vi "control_thor_z825b.vi"() -> ()   [LabVIEW 2013]
panel:
  out "error out":errorcluster
  out "pfPosition":sgl
  in  "stop":bool
  in  "serial":i32
  in  "MG17Motor":refnum<k7>(container)
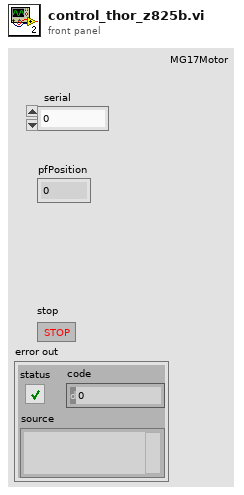
[diagram p1: front panel]
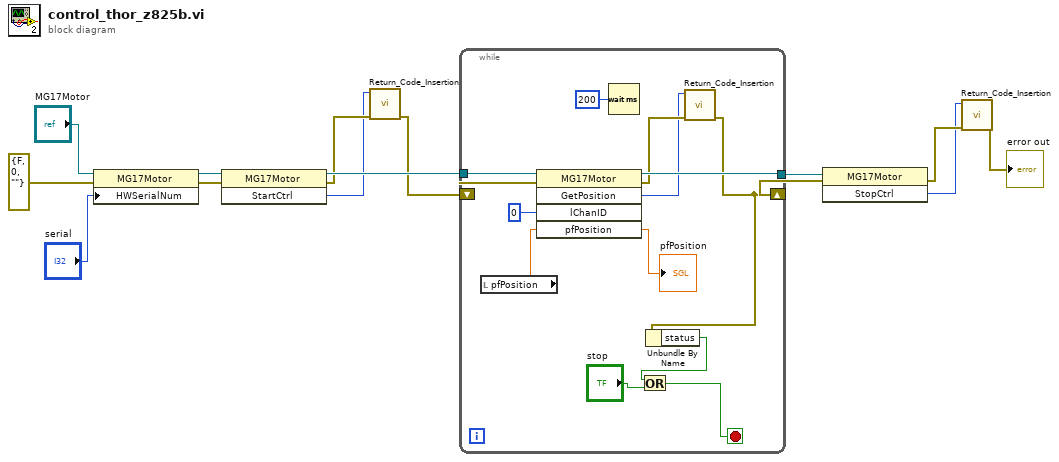
[diagram p0: block diagram]
diagram:
  n1 = property class="MG17Motor"(reference="MG17Motor", error in=errorcluster {"status"=FALSE, "code"=0, "source"=""} ("error in (no error)"), "HWSerialNum"="serial") -> (reference out=w12:refnum<k7>, error out=w8:errorcluster)
  n2 = invoke class="MG17Motor" method="StartCtrl"(reference=w12, error in=w8) -> (reference out=w11:refnum<k7>, error out=w7:errorcluster, "StartCtrl"=w6:i32)  [unwired: 1 in]
  n3 = call "Return_Code_Insertion.vi"("error in (no error)"=w7, "Return Code"=w6) -> ("error out"=w5:errorcluster)  [unwired: 9 in]
  n4 = while {
    tunnel: w11 -> [w27]
    tunnel: [w26] -> w10
    shift-right: [w18] -> w4
    shift-left: w5 -> [w21]
    stop <- w15 stop-if-true
    n5 = local read "pfPosition"() -> (w23:sgl)
    n6 = invoke class="MG17Motor" method="GetPosition"(reference=w27, error in=w21, "lChanID"=0, "pfPosition"=w23) -> (reference out=w26:refnum<k7>, error out=w20:errorcluster, "GetPosition"=w19:i32, "pfPosition"=→"pfPosition":sgl)  [unwired: 1 in, 1 out]
    n7 = Wait (ms)(milliseconds to wait=u32 200) -> ()  [unwired: 1 out]
    n8 = call "Return_Code_Insertion.vi"("error in (no error)"=w20, "Return Code"=w19) -> ("error out"=w18:errorcluster)  [unwired: 9 in]
    n9 = Unbundle By Name(w18) -> ("status"=w17:bool)
    n10 = Or(x=w17, y="stop") -> (x .or. y?=w15:bool)
  }
  n11 = invoke class="MG17Motor" method="StopCtrl"(reference=w10, error in=w4) -> (error out=w3:errorcluster, "StopCtrl"=w2:i32)  [unwired: 1 in, 1 out]
  n12 = call "Return_Code_Insertion.vi"("error in (no error)"=w3, "Return Code"=w2) -> ("error out"=→"error out":errorcluster)  [unwired: 9 in]
